vi "Uninit.vi"(0 "SR865 in":T1, 5 "error in":errorcluster) -> (19 "error out":errorcluster)   [LabVIEW 2018]
uses:
  SR865.ctl
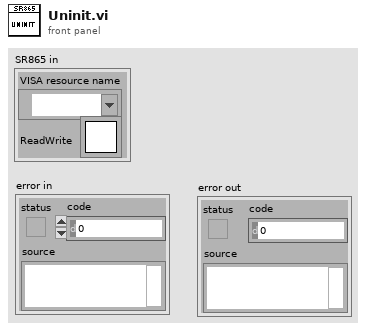
[diagram p1: front panel]
types:
  T1 = typedef "SR865.ctl" = cluster{"VISA resource name":refnum<visa-resource-name>, "ReadWrite":T2}
  T2 = typedef "Semaphore RefNum" = refnum<k1>
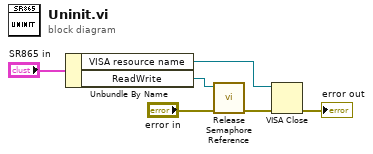
[diagram p0: block diagram]
diagram:
  n1 = Unbundle By Name("SR865 in") -> ("VISA resource name"=w3:refnum<visa-resource-name>, "ReadWrite"=w5:T2)
  n2 = call <vilib>:"Release Semaphore Reference.vi"("error in (no error)"="error in", "semaphore"=w5) -> ("error out"=w2:errorcluster)  [unwired: 8 in, 1 out]
  n3 = VISA Close(VISA resource name=w3, error in (no error)=w2) -> (error out=→"error out":errorcluster)
